vi "Find Speed (Optimized).vi"(0 "[x]":dbl[](array[numeric]), 7 "max window":dbl=1400.0 format="%#_13g", 9 "min window":dbl=45.0 format="%#_13g", 11 "CommSegments":dbl=2.0 format="%#_13g") -> (4 "Speed":dbl)   [LabVIEW 2013]
uses:
  <vilib>/Analysis/2dsp.llb/Power Spectrum (DBL).vi
  <vilib>/Analysis/NI_AALPro.lvlib
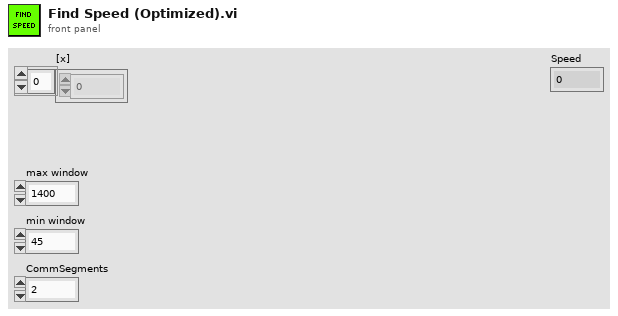
[diagram p1: front panel]
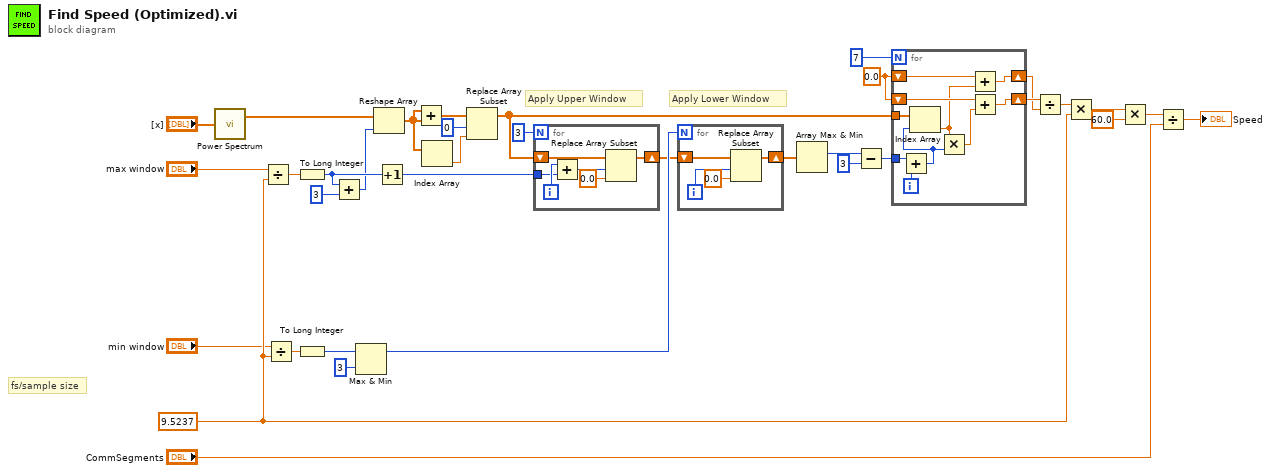
[diagram p0: block diagram]
diagram:
  w32 = 0.0
  w16 = 9.5237 ("df")
  # "fs/sample size"
  # "Apply Lower Window"
  # "Apply Upper Window"
  n1 = call-poly <vilib>:"Power Spectrum.vi"("X"="[x]") -> ("Power Spectrum"=w11:dbl[])  [unwired: 1 out]
  n2 = Divide(x="max window", y=w16) -> (x/y=w12:dbl)
  n3 = Divide(x="min window", y=w16) -> (x/y=w17:dbl)
  n4 = To Long Integer(number=w12) -> (32bit integer=w23:i32)
  n5 = To Long Integer(number=w17) -> (32bit integer=w20:i32)
  n6 = Add(x=w23, y=3) -> (x+y=w18:i32)
  n7 = Max & Min(x=w20, y=3) -> (max(x,y)=w26:i32)  [unwired: 1 out]
  n8 = Reshape Array(w11, w18) -> (w10:dbl[])
  n9 = Increment(x=w23) -> (x+1=w24:i32)
  n10 = Add(x=w10, y=w10) -> (x+y=w9:dbl[])
  n11 = Index Array(array=w10) -> (element=w8:dbl)  [unwired: 1 in]
  n12 = Replace Array Subset(array=w9, new element=w8, index=0) -> (w21:dbl[])
  n13 = for {
    N: 3 -> [_]
    shift-right: [w40] -> w25
    shift-left: w21 -> [w41]
    tunnel: w24 -> [w36]
    i -> [w37]
    n14 = Add(x=w37, y=w36) -> (x+y=w39:i32)
    n15 = Replace Array Subset(array=w41, new element=0.0 ("new element/subarray"), index=w39) -> (w40:dbl[])
  }
  n16 = for {
    N: w26 -> [_]
    shift-right: [w44] -> w27
    shift-left: w25 -> [w45]
    i -> [w42]
    n17 = Replace Array Subset(array=w45, new element=0.0 ("new element/subarray"), index=w42) -> (w44:dbl[])
  }
  n18 = Array Max & Min(array=w27) -> (max index (indices)=w28:i32)  [unwired: 3 out]
  n19 = Subtract(x=w28, y=3) -> (x-y=w31:i32)
  n20 = for {
    N: 7 ("span") -> [_]
    tunnel: w31 -> [w55]
    tunnel: w21 -> [w54]
    shift-right: [w50] -> w33
    shift-left: w32 -> [w51]
    shift-right: [w48] -> w34
    shift-left: w32 -> [w49]
    i -> [w53]
    n21 = Add(x=w55, y=w53) -> (x+y=w52:i32)
    n22 = Index Array(array=w54, index=w52) -> (element=w46:dbl)
    n23 = Multiply(x=w46, y=w52) -> (x*y=w47:dbl)
    n24 = Add(x=w51, y=w46) -> (x+y=w50:dbl)
    n25 = Add(x=w49, y=w47) -> (x+y=w48:dbl)
  }
  n26 = Divide(x=w34, y=w33) -> (x/y=w35:dbl)
  n27 = Multiply(x=w35, y=w16) -> (x*y=w5:dbl)
  n28 = Multiply(x=w5, y=60.0) -> (x*y=w4:dbl)
  n29 = Divide(x=w4, y="CommSegments") -> (x/y=→"Speed":dbl)
